vi "ma_FRF Function FFTin no State.vi"(0 "time signal X":waveform(dbl), 1 "time signal Y":waveform(dbl), 3 "df":dbl, 4 "window":T3=1 items=["Rectangle"=0, "Hanning"=1, "Hamming"=2, "Blackman-Harris"=3, "Exact Blackman"=4, "Blackman"=5, "Flat Top"=6, "4 Term B-Harris "=7, "7 Term B-Harris"=8, "Low Sidelobe"=9, "Blackman Nuttall"=11, "Triangle"=30, "Bartlett-Hanning"=31, "Bohman"=32, "Parzen"=33, "Welch"=34, "Kaiser"=60, "Dolph-Chebyshev"=61, "Gaussian"=62], 5 "view":T1, 7 "error in (no error)":errorcluster, 8 "restart averaging (F)":bool, 9 "averaging parameters":T5={"averaging mode"=enum."No averaging", "weighting mode"=enum."Exponential", "number of averages"=10} {"number of averages" min=1}, 10 "mag-phase":bool, 12 "Sy":cdb[](array[numeric]), 13 "state info":T2 {"Syy" format="%0.2f"; "Sxy" format="%0.2f"; "Sy" format="%0.2f"; "Sxx" format="%0.2f"; "avgs completed" format="%0.2f"; "df" format="%0.2f"; "Sx" format="%0.2f"; "spectrum parameters"."window" items=["Rectangle"=0, "Hanning"=1, "Hamming"=2, "Blackman-Harris"=3, "Exact Blackman"=4, "Blackman"=5, "Flat Top"=6, "4 Term B-Harris "=7, "7 Term B-Harris"=8, "Low Sidelobe"=9, "Blackman Nuttall"=11, "Triangle"=30, "Bartlett-Hanning"=31, "Bohman"=32, "Parzen"=33, "Welch"=34, "Kaiser"=60, "Dolph-Chebyshev"=61, "Gaussian"=62]; "dt" format="%0.2f"; "timestamp" format="%0.2f"; "dt history" format="%0.2f"; "t0 history" format="%0.2f"}, 14 "Sx":cdb[](array[numeric]), 15 "FRF Mode":enum16{"H1", "H2", "H3"}(ring)) -> (16 "averaging done":bool, 17 "state info out":T2 {"Syy" format="%0.2f"; "Sxy" format="%0.2f"; "Sy" format="%0.2f"; "Sxx" format="%0.2f"; "avgs completed" format="%0.2f"; "df" format="%0.2f"; "Sx" format="%0.2f"; "spectrum parameters"."window" items=["Rectangle"=0, "Hanning"=1, "Hamming"=2, "Blackman-Harris"=3, "Exact Blackman"=4, "Blackman"=5, "Flat Top"=6, "4 Term B-Harris "=7, "7 Term B-Harris"=8, "Low Sidelobe"=9, "Blackman Nuttall"=11, "Triangle"=30, "Bartlett-Hanning"=31, "Bohman"=32, "Parzen"=33, "Welch"=34, "Kaiser"=60, "Dolph-Chebyshev"=61, "Gaussian"=62]; "dt" format="%0.2f"; "timestamp" format="%0.2f"; "dt history" format="%0.2f"; "t0 history" format="%0.2f"}, 20 "real or mag":cluster{"f0":dbl, "df":dbl, "real or mag":dbl[]} {"real or mag" format="%.2p"; "f0" format="%0.2p"; "df" format="%0.2p"}, 21 "imag or phase":T4 {"imag or phase" format="%.2p"; "f0" format="%0.2p"; "df" format="%0.2p"}, 24 "coherence":cluster{"f0":dbl, "df":dbl, "coherence":dbl[]}, 25 "averages completed":dbl format="%.2p", 27 "error out":errorcluster)   [LabVIEW 2020, in "NI_MAPro.lvlib"]
doc: "Computes the frequency response and the coherence based on the input signals. Results are returned as <B>real part</B>, <B>imaginary part</B>, and <B>coherence</B>."
uses:
  NI_MAPro.lvlib
  windowTd.ctl
  2-chan State.ctl
  NI_AALPro.lvlib
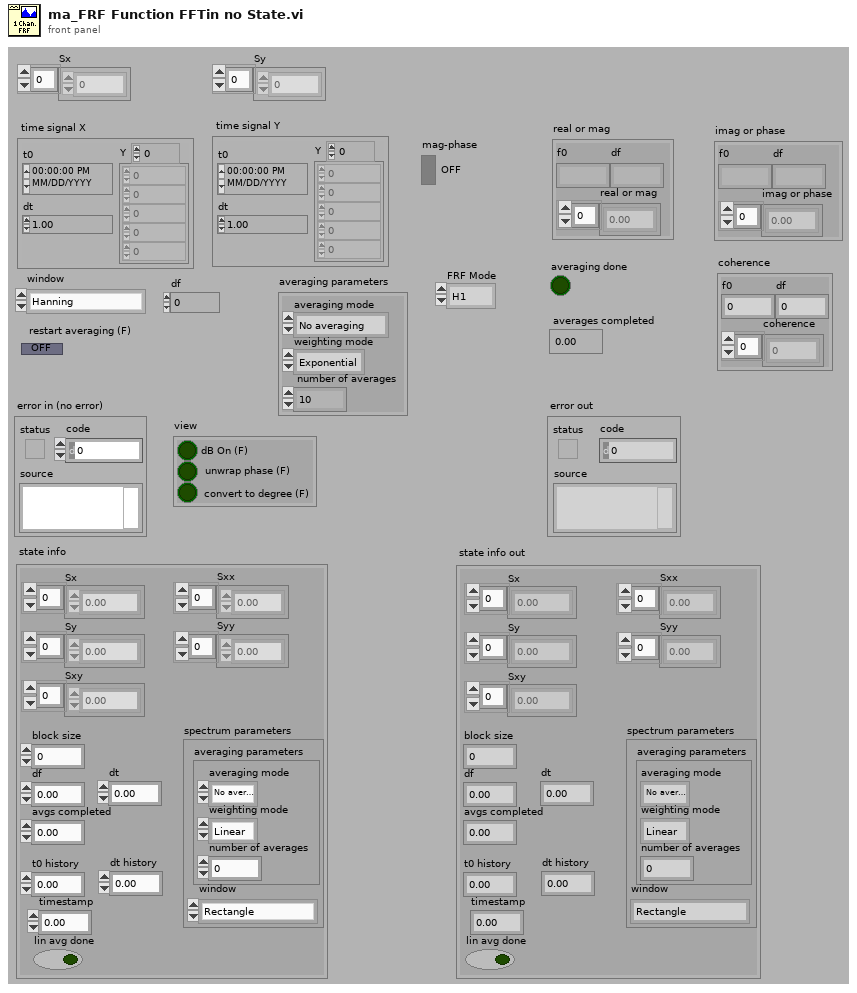
[diagram p1: front panel]
types:
  T1 = cluster{"dB On (F)":bool, "unwrap phase (F)":bool, "convert to degree (F)":bool}
  T2 = typedef "NI_MAPro.lvlib/2-chan State.ctl" = cluster{"Sx":cdb[], "Sy":cdb[], "Sxx":dbl[], "Syy":dbl[], "Sxy":cdb[], "block size":i32, "df":dbl, "dt":dbl, "avgs completed":dbl, "spectrum parameters":cluster{"averaging parameters":cluster{"averaging mode":enum16{"No averaging", "Vector averaging", "RMS averaging", "Peak hold"}, "weighting mode":enum16{"Linear", "Exponential"}, "number of averages":u32}, "window":T3}, "lin avg done":bool, "t0 history":dbl, "dt history":dbl, "timestamp":dbl}
  T3 = typedef "NI_AALPro.lvlib/windowTd.ctl" = u32
  T4 = cluster{"f0":dbl, "df":dbl, "imag or phase":dbl[]}
  T5 = cluster{"averaging mode":enum16{"No averaging", "Vector averaging", "RMS averaging", "Peak hold"}, "weighting mode":enum16{"Linear", "Exponential"}, "number of averages":u32}
  T6 = enum16{"FFT spectrum", "Power spectrum", "Cross spectrum", "Frequency response"}
  T7 = enum16{"No averaging", "Vector averaging", "RMS averaging", "Peak hold"}
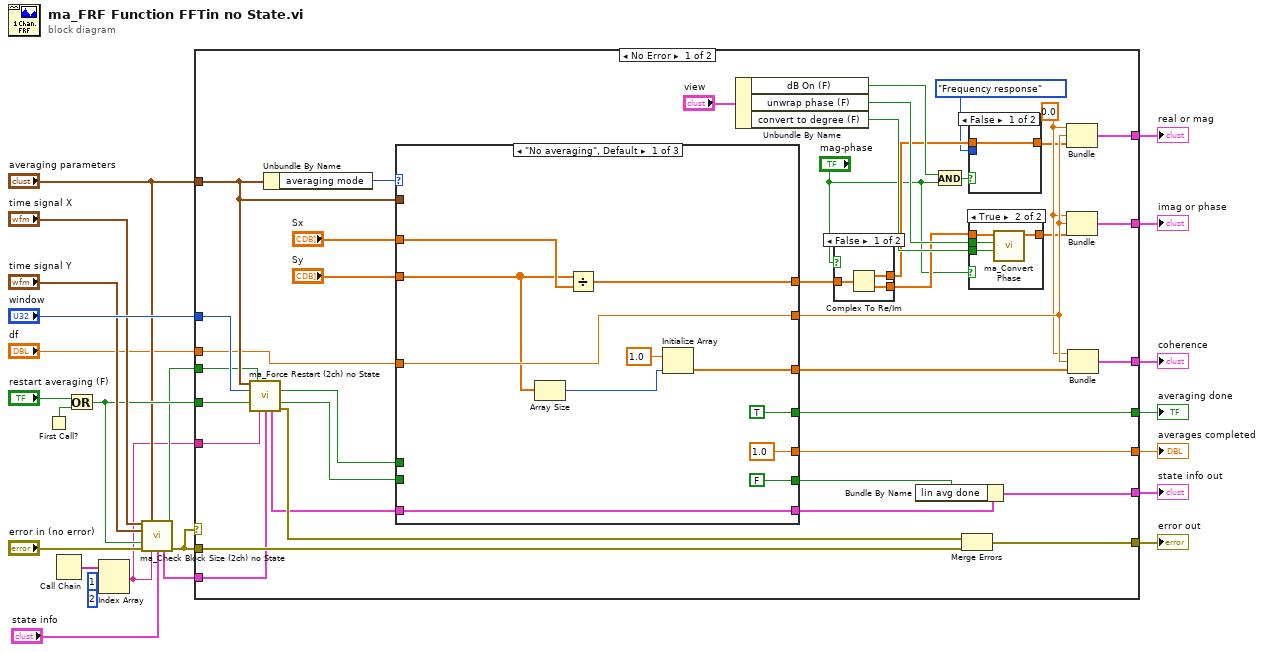
[diagram p0: block diagram]
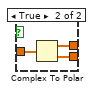
[diagram p2: hidden frame]
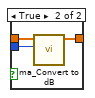
[diagram p4: hidden frame]
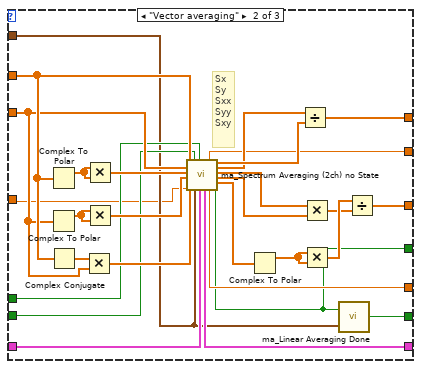
[diagram p5: hidden frame]
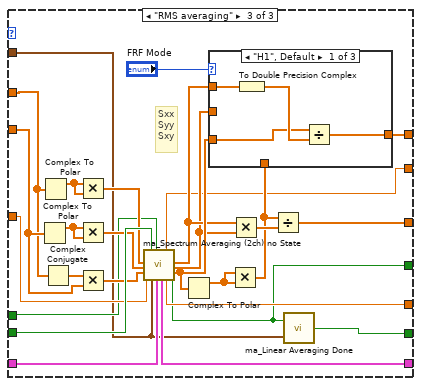
[diagram p6: hidden frame]
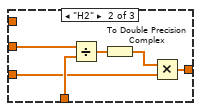
[diagram p7: hidden frame]
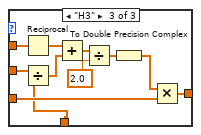
[diagram p8: hidden frame]
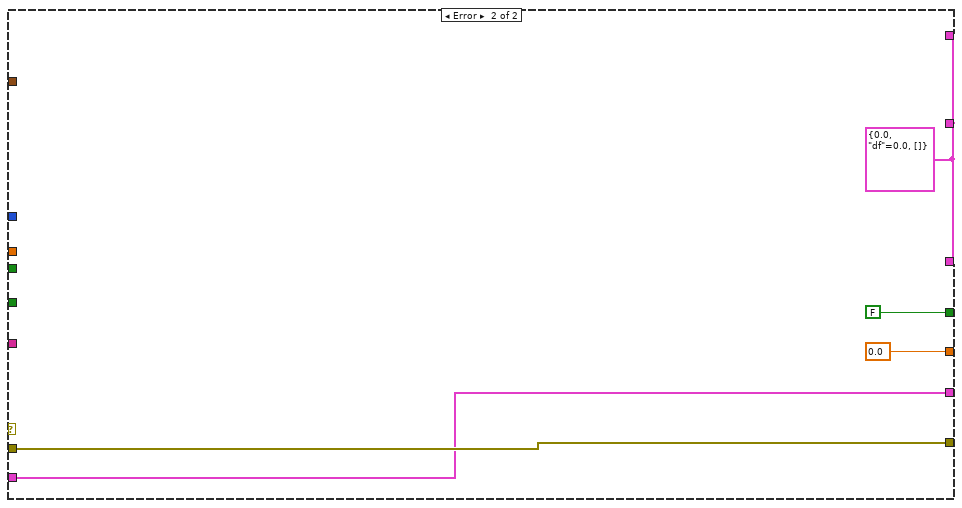
[diagram p9: hidden frame]
diagram:
  n1 = First Call?() -> (First Call?: T/F=w21:bool)
  n2 = Call Chain() -> (call chain=w6:string[])
  n3 = Or(x="restart averaging (F)", y=w21) -> (x .or. y?=w17:bool)
  n4 = Index Array(array=w6, index #1=1 ("Index"), index #2=2 ("Index")) -> (element #1=w5:string)  [unwired: 1 out]
  n5 = call "ma_Check Block Size (2ch) no State.vi"("time signal X"="time signal X", "averaging parameters"="averaging parameters", "time signal Y"="time signal Y", "restart averaging (F)"=w17, "error in"="error in (no error)", "caller VI name"=w5, "state info"="state info") -> ("force restart averaging"=w9:bool, "state info out"=w3:T2, "error out"=w14:errorcluster)  [unwired: 6 out]
  n6 = case shown="No Error" w14 {
    tunnel: [w63 0.0 ("averages completed")] -> w24
    tunnel: [w62 FALSE ("averaging done")] -> w23
    tunnel: "averaging parameters" -> [w61 _]
    tunnel: "window" -> [w60 _]
    tunnel: w17 -> [w59 _]
    tunnel: [w52 w170] -> w15
    tunnel: w14 -> [w50 w170]
    tunnel: [w58 w168] -> w12
    tunnel: [w57 w168] -> w11
    tunnel: [w53 w168] -> w10
    tunnel: w5 -> [w49 _]
    tunnel: w9 -> [w48 _]
    tunnel: w3 -> [w47 w166]
    tunnel: [w41 w166] -> w2
    tunnel: "df" -> [w27 _]
    frame No Error {
      w54 = 0.0
      n7 = call "ma_Force Restart (2ch) no State.vi"("averaging parameters"=w61, "force restart averaging in"=w48, "window"=w60, "restart averaging (F)"=w59, "caller VI name"=w49, "state info"=w47) -> ("force restart averaging"=w45:bool, "retrieve last spectrum"=w44:bool, "state info out"=w43:T2, "error out"=w51:errorcluster)  [unwired: 1 in, 5 out]
      n8 = Unbundle By Name(w61) -> ("averaging mode"=w46:T7)
      n9 = case shown="\"No averaging\", Default" w46 {
        tunnel: [w84 w97 w120] -> w55
        tunnel: w45 -> [_ w98 w125]
        tunnel: w61 -> [_ w91 w118]
        tunnel: [1.0 ("averages completed") w99 w130] -> w63
        tunnel: [w88 w112 w143] -> w56
        tunnel: [TRUE ("averaging done") w96 w121] -> w62
        tunnel: w44 -> [_ w92 w131]
        tunnel: [FALSE ("linear averaging done") w114 w142] -> w42
        tunnel: "Sx" -> [w83 w109 w137]
        tunnel: "Sy" -> [w79 w108 w138]
        tunnel: w27 -> [w84 w90 w126]
        tunnel: w43 -> [w82 w95 w133]
        tunnel: [w82 w94 w132] -> w40
        tunnel: [w81 w93 w119] -> w32
        frame "No averaging", Default {
          n10 = Array Size(array=w79) -> (size(s)=w80:i32)
          n11 = Divide(x=w79, y=w83) -> (x/y=w81:cdb[])
          n12 = Initialize Array(1.0, w80) -> (w88:dbl[])
        }
        frame "Vector averaging" {
          # "Sx\nSy\nSxx\nSyy\nSxy"
          n13 = Complex To Polar(r * e^(i*theta)=w109) -> (r=w111:dbl[])  [unwired: 1 out]
          n14 = Complex To Polar(r * e^(i*theta)=w108) -> (r=w110:dbl[])  [unwired: 1 out]
          n15 = Complex Conjugate(1:w109) -> (0:w113:cdb[])
          n16 = Multiply(x=w113, y=w108) -> (x*y=w105:cdb[])
          n17 = Multiply(x=w111, y=w111) -> (x*y=w107:dbl[])
          n18 = Multiply(x=w110, y=w110) -> (x*y=w106:dbl[])
          n19 = call "ma_Spectrum Averaging (2ch) no State.vi"("Sx"=w109, "Sy"=w108, "Sxx"=w107, "Syy"=w106, "Sxy"=w105, "df"=w90, "retrieve last spectrum (F)"=w92, "averaging parameters"=w91, "restart averaging (F)"=w98, "state info"=w95) -> ("state info out"=w94:T2, "df"=w97:dbl, "averages completed"=w99:dbl, "avg Sx"=w104:cdb[], "avg Sy"=w103:cdb[], "avg Sxx"=w102:dbl[], "avg Syy"=w101:dbl[], "avg Sxy"=w100:cdb[], "averaging done"=w96:bool)  [unwired: 1 in]
          n20 = Complex To Polar(r * e^(i*theta)=w100) -> (r=w115:dbl[])  [unwired: 1 out]
          n21 = Divide(x=w103, y=w104) -> (x/y=w93:cdb[])
          n22 = Multiply(x=w102, y=w101) -> (x*y=w116:dbl[])
          n23 = Multiply(x=w115, y=w115) -> (x*y=w117:dbl[])
          n24 = call "ma_Linear Averaging Done.vi"("averaging parameters"=w91, "averaging done"=w96) -> ("linear averaging done"=w114:bool)
          n25 = Divide(x=w117, y=w116) -> (x/y=w112:dbl[])
        }
        frame "RMS averaging" {
          # "Sxx\nSyy\nSxy"
          n26 = Complex To Polar(r * e^(i*theta)=w138) -> (r=w139:dbl[])  [unwired: 1 out]
          n27 = Complex To Polar(r * e^(i*theta)=w137) -> (r=w140:dbl[])  [unwired: 1 out]
          n28 = Complex Conjugate(1:w137) -> (0:w141:cdb[])
          n29 = Multiply(x=w140, y=w140) -> (x*y=w129:dbl[])
          n30 = Multiply(x=w139, y=w139) -> (x*y=w128:dbl[])
          n31 = Multiply(x=w141, y=w138) -> (x*y=w127:cdb[])
          n32 = call "ma_Spectrum Averaging (2ch) no State.vi"("Sxx"=w129, "Syy"=w128, "Sxy"=w127, "df"=w126, "retrieve last spectrum (F)"=w131, "averaging parameters"=w118, "restart averaging (F)"=w125, "state info"=w133) -> ("state info out"=w132:T2, "df"=w120:dbl, "averages completed"=w130:dbl, "avg Sxx"=w123:dbl[], "avg Syy"=w122:dbl[], "avg Sxy"=w124:cdb[], "averaging done"=w121:bool)  [unwired: 3 in, 2 out]
          n33 = Complex To Polar(r * e^(i*theta)=w124) -> (r=w135:dbl[])  [unwired: 1 out]
          n34 = Multiply(x=w135, y=w135) -> (x*y=w136:dbl[])
          n35 = case shown="\"H1\", Default" "FRF Mode" {
            tunnel: w123 -> [w148 _ w157]
            tunnel: [w147 w153 w158] -> w119
            tunnel: w122 -> [_ w152 w156]
            tunnel: w124 -> [w145 w149 w159]
            tunnel: w136 -> [_ w151 w155]
            frame "H1", Default {
              n36 = To Double Precision Complex(1:w148) -> (0:w146:cdb[])
              n37 = Divide(x=w145, y=w146) -> (x/y=w147:cdb[])
            }
            frame "H2" {
              n38 = Divide(x=w152, y=w151) -> (x/y=w154:dbl[])
              n39 = To Double Precision Complex(1:w154) -> (0:w150:cdb[])
              n40 = Multiply(x=w150, y=w149) -> (x*y=w153:cdb[])
            }
            frame "H3" {
              n41 = Reciprocal(x=w157) -> (1/x=w160:dbl[])
              n42 = Divide(x=w156, y=w155) -> (x/y=w161:dbl[])
              n43 = Add(x=w160, y=w161) -> (x+y=w162:dbl[])
              n44 = Divide(x=w162, y=2.0) -> (x/y=w164:dbl[])
              n45 = To Double Precision Complex(1:w164) -> (0:w165:cdb[])
              n46 = Multiply(x=w165, y=w159) -> (x*y=w158:cdb[])
            }
          }
          n47 = Multiply(x=w123, y=w122) -> (x*y=w144:dbl[])
          n48 = Divide(x=w136, y=w144) -> (x/y=w143:dbl[])
          n49 = call "ma_Linear Averaging Done.vi"("averaging parameters"=w118, "averaging done"=w121) -> ("linear averaging done"=w142:bool)
        }
      }
      n50 = Unbundle By Name("view") -> ("dB On (F)"=w36:bool, "unwrap phase (F)"=w35:bool, "convert to degree (F)"=w34:bool)
      n51 = case shown="False" "mag-phase" {
        tunnel: w32 -> [w66 w69]
        tunnel: [w65 w68] -> w31
        tunnel: [w64 w67] -> w30
        frame False {
          n52 = Complex To Re/Im(x + iy=w66) -> (x=w65:dbl[], y=w64:dbl[])
        }
        frame True {
          n53 = Complex To Polar(r * e^(i*theta)=w69) -> (r=w68:dbl[], theta=w67:dbl[])
        }
      }
      n54 = Bundle By Name(cluster=w40, "lin avg done"=w42) -> (w41:T2)
      n55 = And(x=w36, y="mag-phase") -> (x .and. y?=w37:bool)
      n56 = Merge Errors(w51, w50) -> (w52:errorcluster)
      n57 = case shown="False" w37 {
        tunnel: [w75 w77] -> w38
        tunnel: w31 -> [w75 w78]
        tunnel: T6."Frequency response" ("spectrum type") -> [_ w76]
        frame False {
        }
        frame True {
          n58 = call "ma_Convert to dB.vi"("spectrum type"=w76, "spectrum"=w78) -> ("spectrum in dB"=w77:dbl[])  [unwired: 9 out]
        }
      }
      n59 = case shown="True" "mag-phase" {
        tunnel: [w70 w71] -> w33
        tunnel: w30 -> [w70 w74]
        tunnel: w35 -> [_ w73]
        tunnel: w34 -> [_ w72]
        frame False {
        }
        frame True {
          n60 = call "ma_Convert Phase.vi"("convert to degree (F)"=w72, "unwrap phase (F)"=w73, "phase (radian)"=w74) -> ("scaled phase"=w71:dbl[])  [unwired: 3 in, 5 out]
        }
      }
      n61 = Bundle(w54, "df"=w55, "spectrum in dB"=w38) -> (w58:cluster{dbl, "df":dbl, "spectrum in dB":dbl[]})  [unwired: 1 out]
      n62 = Bundle(w54, "df"=w55, "scaled phase"=w33) -> (w57:cluster{dbl, "df":dbl, "scaled phase":dbl[]})  [unwired: 1 out]
      n63 = Bundle(w54, "df"=w55, w56) -> (w53:cluster{dbl, "df":dbl, dbl[]})  [unwired: 1 out]
    }
    frame Error {
      w168 = cluster{dbl, "df":dbl, dbl[]} {0.0, "df"=0.0, []}
    }
  }
  "averages completed" <- w24
  "error out" <- w15
  "averaging done" <- w23
  "coherence" <- w10
  "imag or phase" <- w11
  "real or mag" <- w12
  "state info out" <- w2
